vi "Cluster Elements.vi"(8 "error in (no error)":errorcluster, 11 "Cluster Variant":variant) -> (0 "error out":errorcluster, 3 "Cluster Elements":variant[](array[variant]))   [LabVIEW 2013, in "LV JSON.lvlib"]
doc: "Get elements of cluster."
uses:
  LV JSON.lvlib
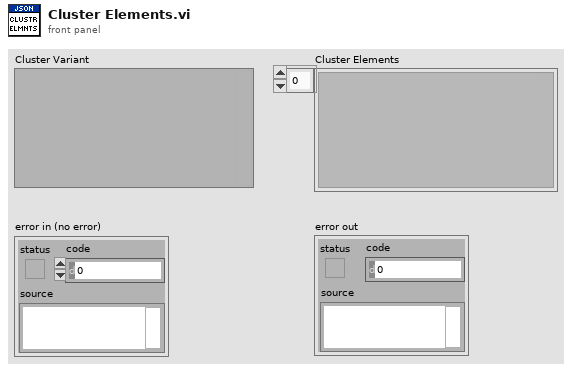
[diagram p1: front panel]
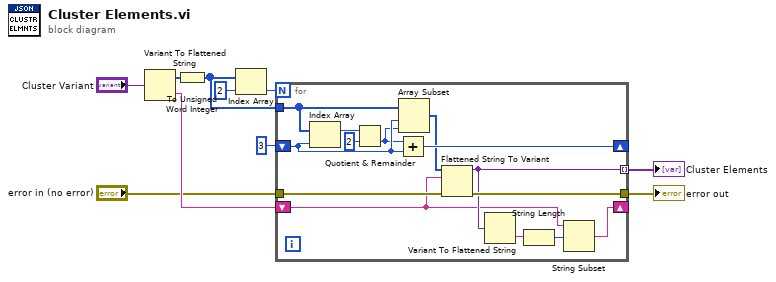
[diagram p0: block diagram]
diagram:
  n1 = Variant To Flattened String(Variant="Cluster Variant") -> (data string=w10:string, 1:w8:i16[])
  n2 = To Unsigned Word Integer(number=w8) -> (unsigned 16bit integer=w7:u16[])
  n3 = Index Array(array=w7, index=2) -> (element=w3:u16)
  n4 = for {
    N: w3 -> [_]
    shift-right: [w23] -> _
    shift-left: 3 ("Index") -> [w22]
    tunnel: w7 -> [w24]
    tunnel: "error in (no error)" -> [w17]
    tunnel: [w16] -> w2
    tunnel: [w14] -> w1 mode=indexing
    shift-right: [w12] -> _
    shift-left: w10 -> [w11]
    n5 = Index Array(array=w24, index=w22) -> (element=w20:u16)
    n6 = Quotient & Remainder(x=w20, y=i16 2) -> (floor(x/y)=w21:u16)  [unwired: 1 out]
    n7 = Add(x=w21, y=w22) -> (x+y=w23:i32)
    n8 = Array Subset(array=w24, index=w22, length=w21) -> (w18:u16[])
    n9 = Flattened String To Variant(4:w17, 6:w11, 7:w18) -> (0:w16:errorcluster, 3:w14:variant)
    n10 = Variant To Flattened String(Variant=w14) -> (data string=w15:string)  [unwired: 1 out]
    n11 = String Length(string=w15) -> (length=w13:i32)
    n12 = String Subset(string=w11, offset (0)=w13) -> (substring=w12:string)  [unwired: 1 out]
  }
  "error out" <- w2
  "Cluster Elements" <- w1
